vi "Task_Enum.vi"(8 "error in (no error)":errorcluster caption="错误输入（无错误）", 10 "Enum":T1(ring), 11 "ParentActor输入":refnum<class "ParentActor.lvclass">) -> (0 "error out":errorcluster caption="错误输出", 3 "ParentActor输出":refnum<class "ParentActor.lvclass">)   [LabVIEW 2014, in "UnitTest.lvlib" / "ParentActor.lvclass"]
uses:
  ParentActor.lvclass
  labview/1603/zsRobotSynergeticSystem/zsLib/zsActor/zsActor.lvclass
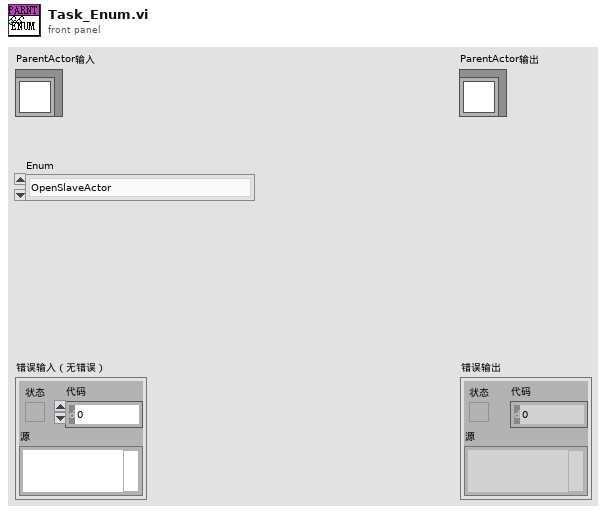
[diagram p1: front panel]
types:
  T1 = enum16{"OpenSlaveActor", "Idle", "StopSlaveActor"}
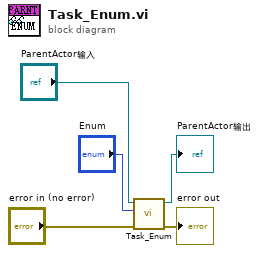
[diagram p0: block diagram]
diagram:
  n1 = call-parent "Task_Enum.vi"("error in (no error)"="error in (no error)", "Enum"="Enum", "zsActor输入"="ParentActor输入") -> ("error out"=→"error out":errorcluster, "zsActor输出"=→"ParentActor输出":refnum<class "ParentActor.lvclass">)  [unwired: 7 in]
